vi "init.vi"(8 "error in (no error)":errorcluster) -> (0 "error out":errorcluster)   [LabVIEW 2010]
uses:
  Variables/GlobalSetCamerasOnOff.vi
panel:
  in  "TemperatureIn":T1
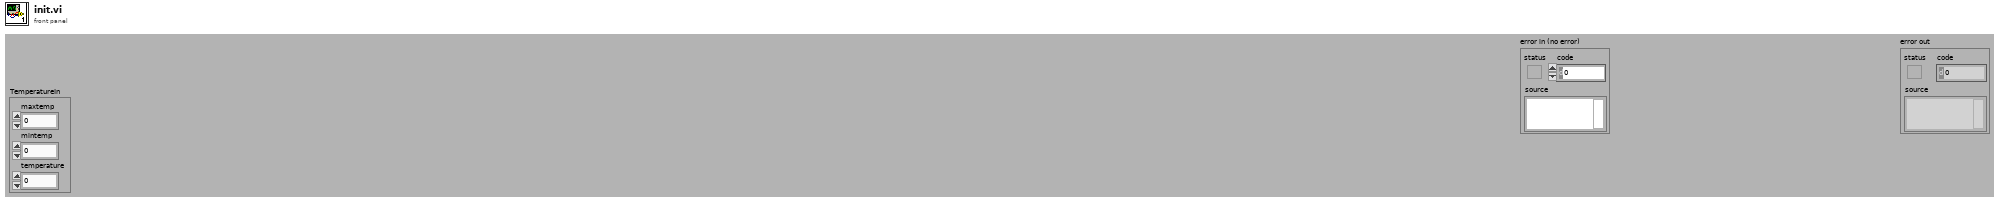
[diagram p1: front panel]
types:
  T1 = cluster{"maxtemp":i32, "mintemp":i32, "temperature":i32}
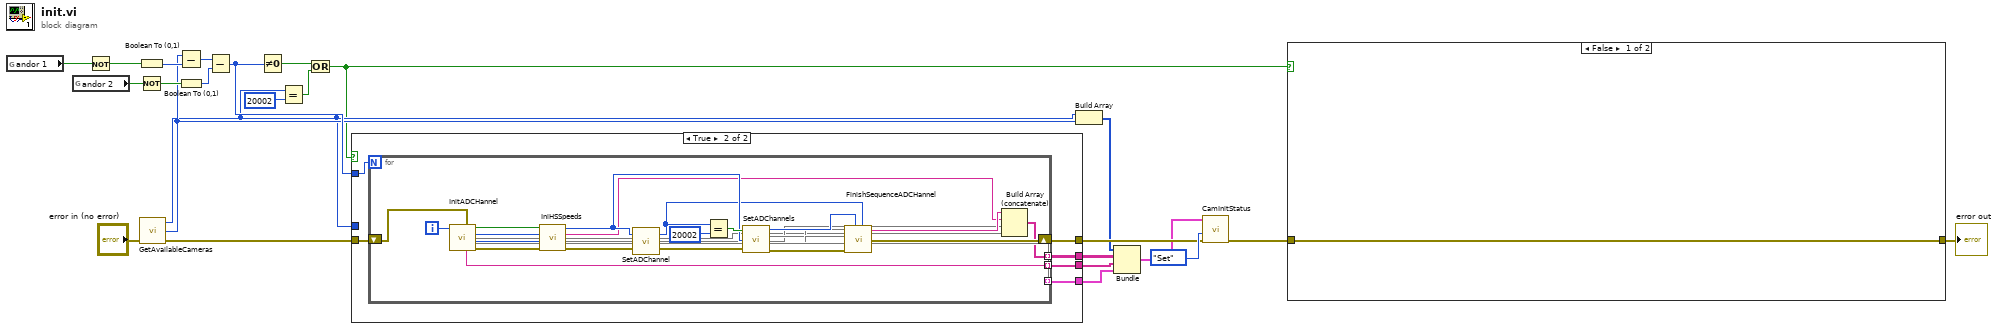
[diagram p0: block diagram]
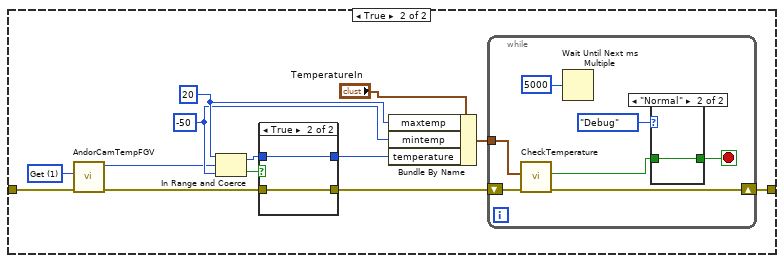
[diagram p2: hidden frame]
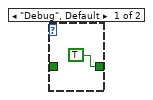
[diagram p3: hidden frame]
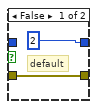
[diagram p4: hidden frame]
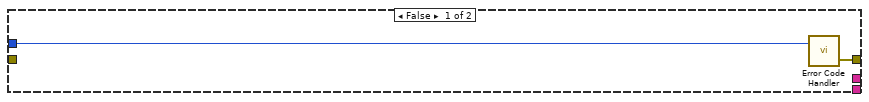
[diagram p5: hidden frame]
diagram:
  n1 = global read "GlobalSetCamerasOnOff.vi" "andor 1"() -> (w6:bool)
  n2 = global read "GlobalSetCamerasOnOff.vi" "andor 2"() -> (w5:bool)
  n3 = Not(x=w6) -> (.not. x?=w18:bool)
  n4 = Boolean To (0,1)(Boolean=w18) -> (0, 1=w20:i16)
  n5 = Not(x=w5) -> (.not. x?=w19:bool)
  n6 = call "GetAvailableCameras.vi"("error in (no error)"="error in (no error)") -> ("error out"=w4:errorcluster, "totalCameras"=w13:i32, "DLL error code"=w12:u32)  [unwired: 2 in]
  n7 = Subtract(x=w13, y=w20) -> (x-y=w21:i32)
  n8 = Boolean To (0,1)(Boolean=w19) -> (0, 1=w22:i16)
  n9 = Subtract(x=w21, y=w22) -> (x-y=w17:i32)
  n10 = Not Equal To 0?(x=w17) -> (x != 0?=w23:bool)
  n11 = Equal?(x=w12, y=u32 20002) -> (x = y?=w24:bool)
  n12 = Or(x=w23, y=w24) -> (x .or. y?=w1:bool)
  n13 = case shown="True" w1 {
    tunnel: w4 -> [_ w32]
    tunnel: w12 -> [w27 _]
    tunnel: [w26 w33] -> w14
    tunnel: w17 -> [_ w31]
    tunnel: [_ w30] -> w9
    tunnel: [_ w29] -> w10
    tunnel: [_ w28] -> w11
    frame False {
      n14 = call "Error Code Handler.vi"("DLL error code"=w27) -> ("error out"=w26:errorcluster)  [unwired: 1 in, 1 out]
    }
    frame True {
      n15 = for {
        N: w31 -> [_]
        shift-right: [w48] -> w33
        shift-left: w32 -> [w55]
        tunnel: [w34] -> w30 mode=indexing
        tunnel: [w36] -> w29 mode=indexing
        tunnel: [w44] -> w28 mode=indexing
        i -> [w35]
        n16 = call "InitADCHannel.vi"("error out"=w55, 6:w35) -> ("Boolean"=w57:bool, "number"=w47:i32, "DLL error code"=w45:u32, "String"=w36:string, "error out 2"=w56:errorcluster, 7:w37, 8:w44)
        n17 = call "IniHSSpeeds.vi"("error out 2"=w56, "DLL error code"=w45, "number"=w47, "Boolean"=w57) -> ("error out"=w49:errorcluster, 1:w38, "to shell"=w39:string, "Numeric"=w46:i32)
        n18 = call "SetADChannel.vi"("error in (no error)"=w49, "channel"=w46) -> ("error out"=w52:errorcluster, "DLL error code"=w41:u32)
        n19 = Equal?(x=w41, y=u32 20002) -> (x = y?=w51:bool)
        n20 = call "SetADChannels.vi"("error out"=w52, "Numeric"=w46, "Boolean"=w51) -> ("error out 2"=w54:errorcluster, 4:w43, 5:w42, "Numeric 2"=w53:i32)
        n21 = call "FinishSequenceADCHannel.vi"(1:w41, "Numeric 2"=w53, 6:w42, 7:w43, "error out 2"=w54) -> ("to shell"=w40:string, "error out"=w48:errorcluster)  [unwired: 4 in]
        n22 = Build Array (concatenate)(w40, w39, w38, w37) -> (w34:string[])
      }
    }
  }
  n23 = Build Array(w12, w13) -> (w8:u32[])
  n24 = Bundle(w8, w9, w10, w11) -> (w7:cluster{u32[], string[][], string[], void})  [unwired: 1 in]
  n25 = call "CamInitStatus.vi"("error in"=w14, "Set_Get"=enum16{"Set", "Get"}."Set", "CamValsInit set"=w7) -> ("error out"=w3:errorcluster)  [unwired: 7 in, 1 out]
  n26 = case shown="False" w1 {
    tunnel: w3 -> [w58 w60]
    tunnel: [w58 w59] -> w2
    frame False {
    }
    frame True {
      w64 = u16 1 items=["Set", "Get"] ("Set_Get")
      w67 = -50 ("mintemp")
      w68 = 20 ("maxtemp")
      n27 = call "AndorCamTempFGV.vi"("error in"=w60, "Set_Get"=w64) -> ("error out"=w62:errorcluster, "TempOut"=w63:i32)  [unwired: 8 in]
      n28 = In Range and Coerce(upper limit=w68, x=w63, lower limit=w67) -> (coerced(x)=w65:i32, In Range?=w66:bool)
      n29 = case shown="True" w66 {
        tunnel: [2 ("mintemp") w84] -> w69
        tunnel: w65 -> [_ w84]
        tunnel: w62 -> [w81 w83]
        tunnel: [w81 w83] -> w61
        frame False {
          # "default"
        }
        frame True {
        }
      }
      n30 = Bundle By Name(cluster="TemperatureIn", "maxtemp"=w68, "mintemp"=w67, "temperature"=w69) -> (w70:T1)
      n31 = while {
        tunnel: w70 -> [w78]
        shift-right: [w75] -> w59
        shift-left: w61 -> [w77]
        stop <- w73 stop-if-true
        n32 = call "CheckTemperature.vi"("error in (no error)"=w77, 10:w78) -> ("error out"=w75:errorcluster, "TemperatureReached"=w72:bool)  [unwired: 7 in, 1 out]
        n33 = Wait Until Next ms Multiple(millisecond multiple=u32 5000) -> ()  [unwired: 1 out]
        n34 = case shown="\"Normal\"" enum16{"Debug", "Normal"}."Debug" {
          tunnel: [TRUE w80] -> w73
          tunnel: w72 -> [_ w80]
          frame "Debug", Default {
          }
          frame "Normal" {
          }
        }
      }
    }
  }
  "error out" <- w2
